vi "RT main.vi"() -> ()   [LabVIEW 2017]
doc: "This example demonstrates how to acquire a continuous amount of data (Waveform) using the DAQ device's internal clock. It also shows how to synchronize two devices for different device families (E Series, S Series, M Series, X Series, DSA, and SC Express), to simultaneously acquire the data.\n\nFor instructions on how to connect your signals to the DAQ device, refer to your device documentation."
uses:
  <vilib>/addons/_NISVFA/_Shared subVIs/Controls/svc_Engineering Units Text Ring.ctl
  <vilib>/addons/_NISVFA/_Shared subVIs/Controls/svc_Weighting Filter Text Ring.ctl
  typedefs/Data.ctl
  <vilib>/Utility/error.llb/DialogType.ctl
  <vilib>/DAQmx/read.llb/DAQmx Read (Analog 1D Wfm NChan NSamp).vi
  <vilib>/Analysis/baseanly.llb/Mean (DBL).vi
  <vilib>/DAQmx/read.llb/DAQmx Read (Analog Wfm 1Chan NSamp).vi
  <vilib>/addons/Sound and Vibration/svt_Calibration/SVL Scale Voltage to EU (1 Ch).vi
  <vilib>/DAQmx/read.llb/DAQmx Read (Analog DBL 1Chan 1Samp).vi
  <extravilib>/ChannelInstances/Stream-a[.](bool)/Read With Abort.vi
  <extravilib>/ChannelInstances/Stream-t'Data.ctl'/Read With Abort.vi
  <extravilib>/ChannelInstances/Stream-a[.](bool)/Write With Abort.vi
  <vilib>/addons/_NISVFA/_Shared subVIs/Common/svc_Set SV Channel Info.vi
  <extravilib>/ChannelInstances/Stream-t'Data.ctl'/Write With Abort.vi
  <extravilib>/ChannelInstances/Stream-a[.](bool)/EndpointRead.vi
  <extravilib>/ChannelInstances/Stream-t'Data.ctl'/EndpointRead.vi
  <extravilib>/ChannelInstances/Stream-a[.](bool)/Endpoint.vi
  <vilib>/addons/_NISVFA/_Shared subVIs/Common/svc_Set SV Channel Info (variant).vi
  <extravilib>/ChannelInstances/Stream-t'Data.ctl'/Endpoint.vi
  <vilib>/addons/_NISVFA/_Shared subVIs/Common/SVL Set dB Reference (variant).vi
  <vilib>/DAQmx/create/channels.llb/DAQmx Create Channel (AI-Voltage-Basic).vi
  <vilib>/DAQmx/configure/timing.llb/DAQmx Timing (Sample Clock).vi
  <vilib>/DAQmx/create/channels.llb/DAQmx Create Channel (AI-Temperature-Thermocouple).vi
  <vilib>/httpClient/POSTBuffer.vi
  <extravilib>/ChannelInstances/Stream-a[.](bool)/Instantiate.vi
  <extravilib>/ChannelInstances/Stream-a[.](bool)/)Channel.vi
  <resource>/ChannelSupport/_ChannelSupport/WaitIfNeeded.vi
  <extravilib>/ChannelInstances/Stream-t'Data.ctl'/Instantiate.vi
  <extravilib>/ChannelInstances/Stream-t'Data.ctl'/)Channel.vi
  <vilib>/Skyline/File/File/Send File.vi
  <vilib>/DAQmx/miscellaneous.llb/DAQmx Fill In Error Info.vi
  <vilib>/addons/Sound and Vibration/Order Analysis/Tach Process/OAT Analog Tacho Process (1 Tacho).vi
  <vilib>/addons/_NISVFA/_Shared subVIs/Common/svc_Engineering Units to Unit Label.vi
  <vilib>/addons/_NISVFA/_Shared subVIs/Common/svc_Compute Scale Factor to Convert V to EU.vi
  <vilib>/addons/_NISVFA/_Shared subVIs/Common/svc_Compute Scale Factor to Convert C to EU.vi
  <vilib>/addons/_NISVFA/_Shared subVIs/Common/svc_Set dB ref if Pascal.vi
  <vilib>/addons/_NISVFA/_Shared subVIs/Common/svc_Caller VI Returned in Error Source.vi
  <vilib>/addons/Sound and Vibration/svt_Level/SVL Running RMS Level (1 Ch).vi
  <vilib>/addons/Sound and Vibration/svt_Calibration/SoundVib_Calibration.lvlib
  <vilib>/addons/Sound and Vibration/svt_Level/SoundVib_VibrationLevel.lvlib
  <vilib>/addons/Sound and Vibration/Order Analysis/Tach Process/SoundVib_TachProcess.lvlib
  <vilib>/Analysis/NI_AALBase.lvlib
  <vilib>/httpClient/LabVIEWHTTPClient.lvlib
  <vilib>/NI_Real-Time Target Support.lvlib
  <extravilib>/ChannelInstances/Stream-t'Data.ctl'.lvlib
  <extravilib>/ChannelInstances/Stream-a[.](bool).lvlib
  <vilib>/Skyline/File/File/NI Skyline File.lvclass
panel:
  out "running RMS":dbl=nan format="%.6f"
  out "network disconnected":T1[](array[typedef]) {"RMS" format="%0.6f"; "RPM" format="%0.2f"; "Voltage" format="%0.2f"; "Current" format="%0.2f"; "Temperature" format="%0.2f"}
  in  "Write to TDMS?":bool
  out "network connected":T1 {"RMS" format="%0.6f"; "RPM" format="%0.2f"; "Voltage" format="%0.2f"; "Current" format="%0.2f"; "Temperature" format="%0.2f"}
  out "Y":bool
  in  "Buttoon 1":bool
  in  "Button 2":bool
  in  "Button 3":bool
  in  "Ipad 2":bool
  in  "Ipad 3":bool
  in  "Ipad 1":bool
  out "Valve":bool[](array[boolean])
  out "X":bool
  out "JSON":string
  in  "integration time [s]":dbl=1.0
  out "Temp.":dbl format="%0.2f"
  out "Current":dbl format="%0.2f"
  out "Voltage":dbl format="%0.2f"
  out "RPM mean":dbl format="%0.2f"
  out "Motor Voltage & Current":waveform(dbl)[](graph)
  in  "Vibration Channel Info":T4={"sensor sensitivity"=1000.0, "engineering units"=1, "dB reference"=1.0, "custom label"="EU", "weighting filter"=0, "pregain"=0.0} {"pregain" format="%.2f"; "weighting filter" items=["Linear", "A-weighting", "B-weighting", "C-weighting", "ITU-R 468-4", "Dolby", "CCITT", "C-message", "Wb", "Wc", "Wd", "We", "Wf", "Wh", "Wj", "Wk", "Wm", "AES17 20 kHz lowpass", "AES17 40 kHz lowpass", "AES17 20 kHz highpass", "AES17 40 kHz highpass"]; "dB reference" format="%^.1e"; "engineering units" items=["custom..."=0, "V"=1, "A"=21, "C"=30, "pC"=31, "s"=32, "-"=29, "Pa"=2, "N"=20, "g"=3, "m/s^2"=4, "m/s"=5, "m"=6, "mm/s"=12, "mm"=13, "micron/s"=14, "micron"=15, "in/s^2"=7, "in/s"=8, "in"=9, "mil/s"=10, "mil"=11, "rad/s^2"=16, "rad/s"=17, "rad"=18, "deg/s^2"=26, "deg/s"=27, "deg"=28, "RPM"=22, "cycle/s^2"=23, "Hz"=24, "cycle"=25, "strain"=19]; "sensor sensitivity" format="%#_5f"}
  in  "Acquire Stop":bool
  in  "CJC Value":dbl=25.0 format="%0.2f"
  in  "CJC Source":i32(ring)=10116 items=["Built-In"=10200, "Constant Value"=10116, "Channel"=10113]
  in  "Thermocouple Type":i32(ring)=10073 items=["J"=10072, "K"=10073, "N"=10077, "R"=10082, "S"=10085, "T"=10086, "B"=10047, "E"=10055]
  in  "Units":i32(ring)=10143 items=["Deg C"=10143, "Deg F"=10144, "Kelvins"=10325, "Deg R"=10145, "From Custom Scale"=10065]
  out "Thermocouple waveform":dbl(graph)
  in  "Motor Voltage & Current & RPM Sample":i32=5120
  in  "Motor Voltage & Current & RPM Sample Rate":dbl=25600.0
  in  "Thermocouple":tag="Mod3/ai1"
  out "Vibration":waveform(dbl)(graph)
  in  "Vibration Sample":i32=5120
  in  "Vibration Sample Rate":dbl=25600.0
  in  "Motor Voltage &Current& RPM":tag="Mod2/ai0:2"
  in  "Vibration":tag="Mod1/ai0"
  # "Vibration Settings"
  # "Vibration"
  # "Motor Voltage & Current & RPM"
  # "Motor Voltage & current & RPM Settings"
  # "Temperature"
  # "Tempearture"
  # "Thermocouple Settings"
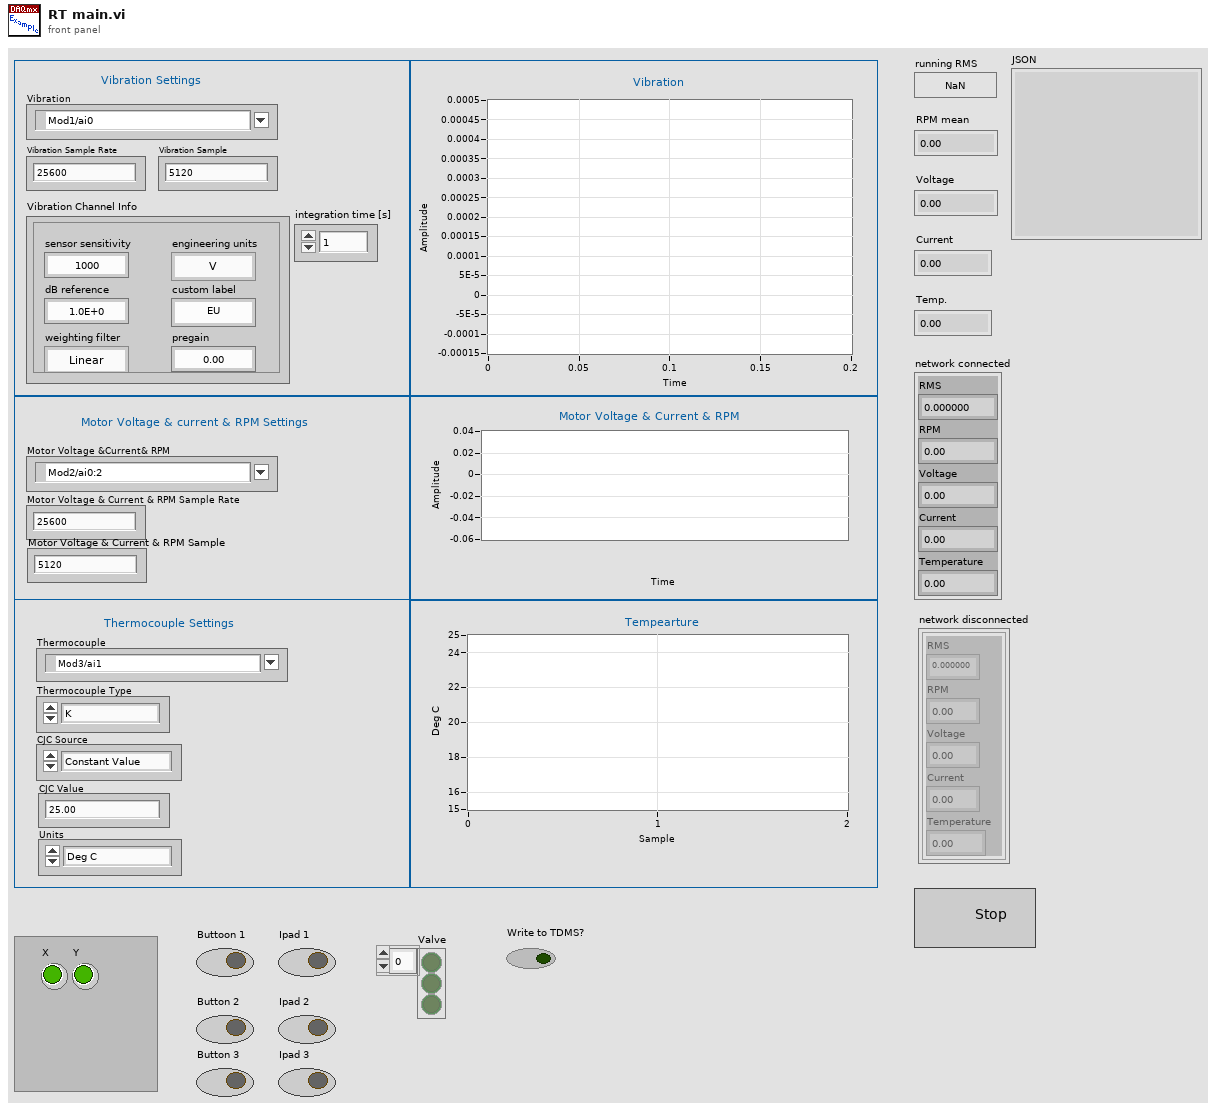
[diagram p1: front panel]
types:
  T1 = typedef "Data.ctl" = cluster{"RMS":dbl, "RPM":dbl, "Voltage":dbl, "Current":dbl, "Temperature":dbl}
  T2 = typedef "svc_Engineering Units Text Ring.ctl" = u16
  T3 = typedef "svc_Weighting Filter Text Ring.ctl" = u16
  T4 = cluster{"sensor sensitivity":dbl, "engineering units":T2, "dB reference":dbl, "custom label":string, "weighting filter":T3, "pregain":dbl}
  T5 = enum16{"open", "open or create", "create or replace", "create", "open (read-only)"}
  T6 = typedef "DialogType.ctl" = u16
  T7 = typedef "SoundVib_TachProcess.lvlib/speed profile.ctl" = cluster{"time [s]":dbl[], "speed [RPM]":dbl[]}
  T8 = typedef "Stream-t'Data.ctl'.lvlib/)Channel.ctl" = refnum<queue>
  T9 = typedef "Stream-a[.](bool).lvlib/)Channel.ctl" = refnum<queue>
  T10 = typedef "LabVIEWHTTPClient.lvlib/ClientHandle.ctl" = refnum<k1>
  T11 = cluster{"RMS":string, "RPM":string, "Voltage":string, "Current":string, "Temperature":string}
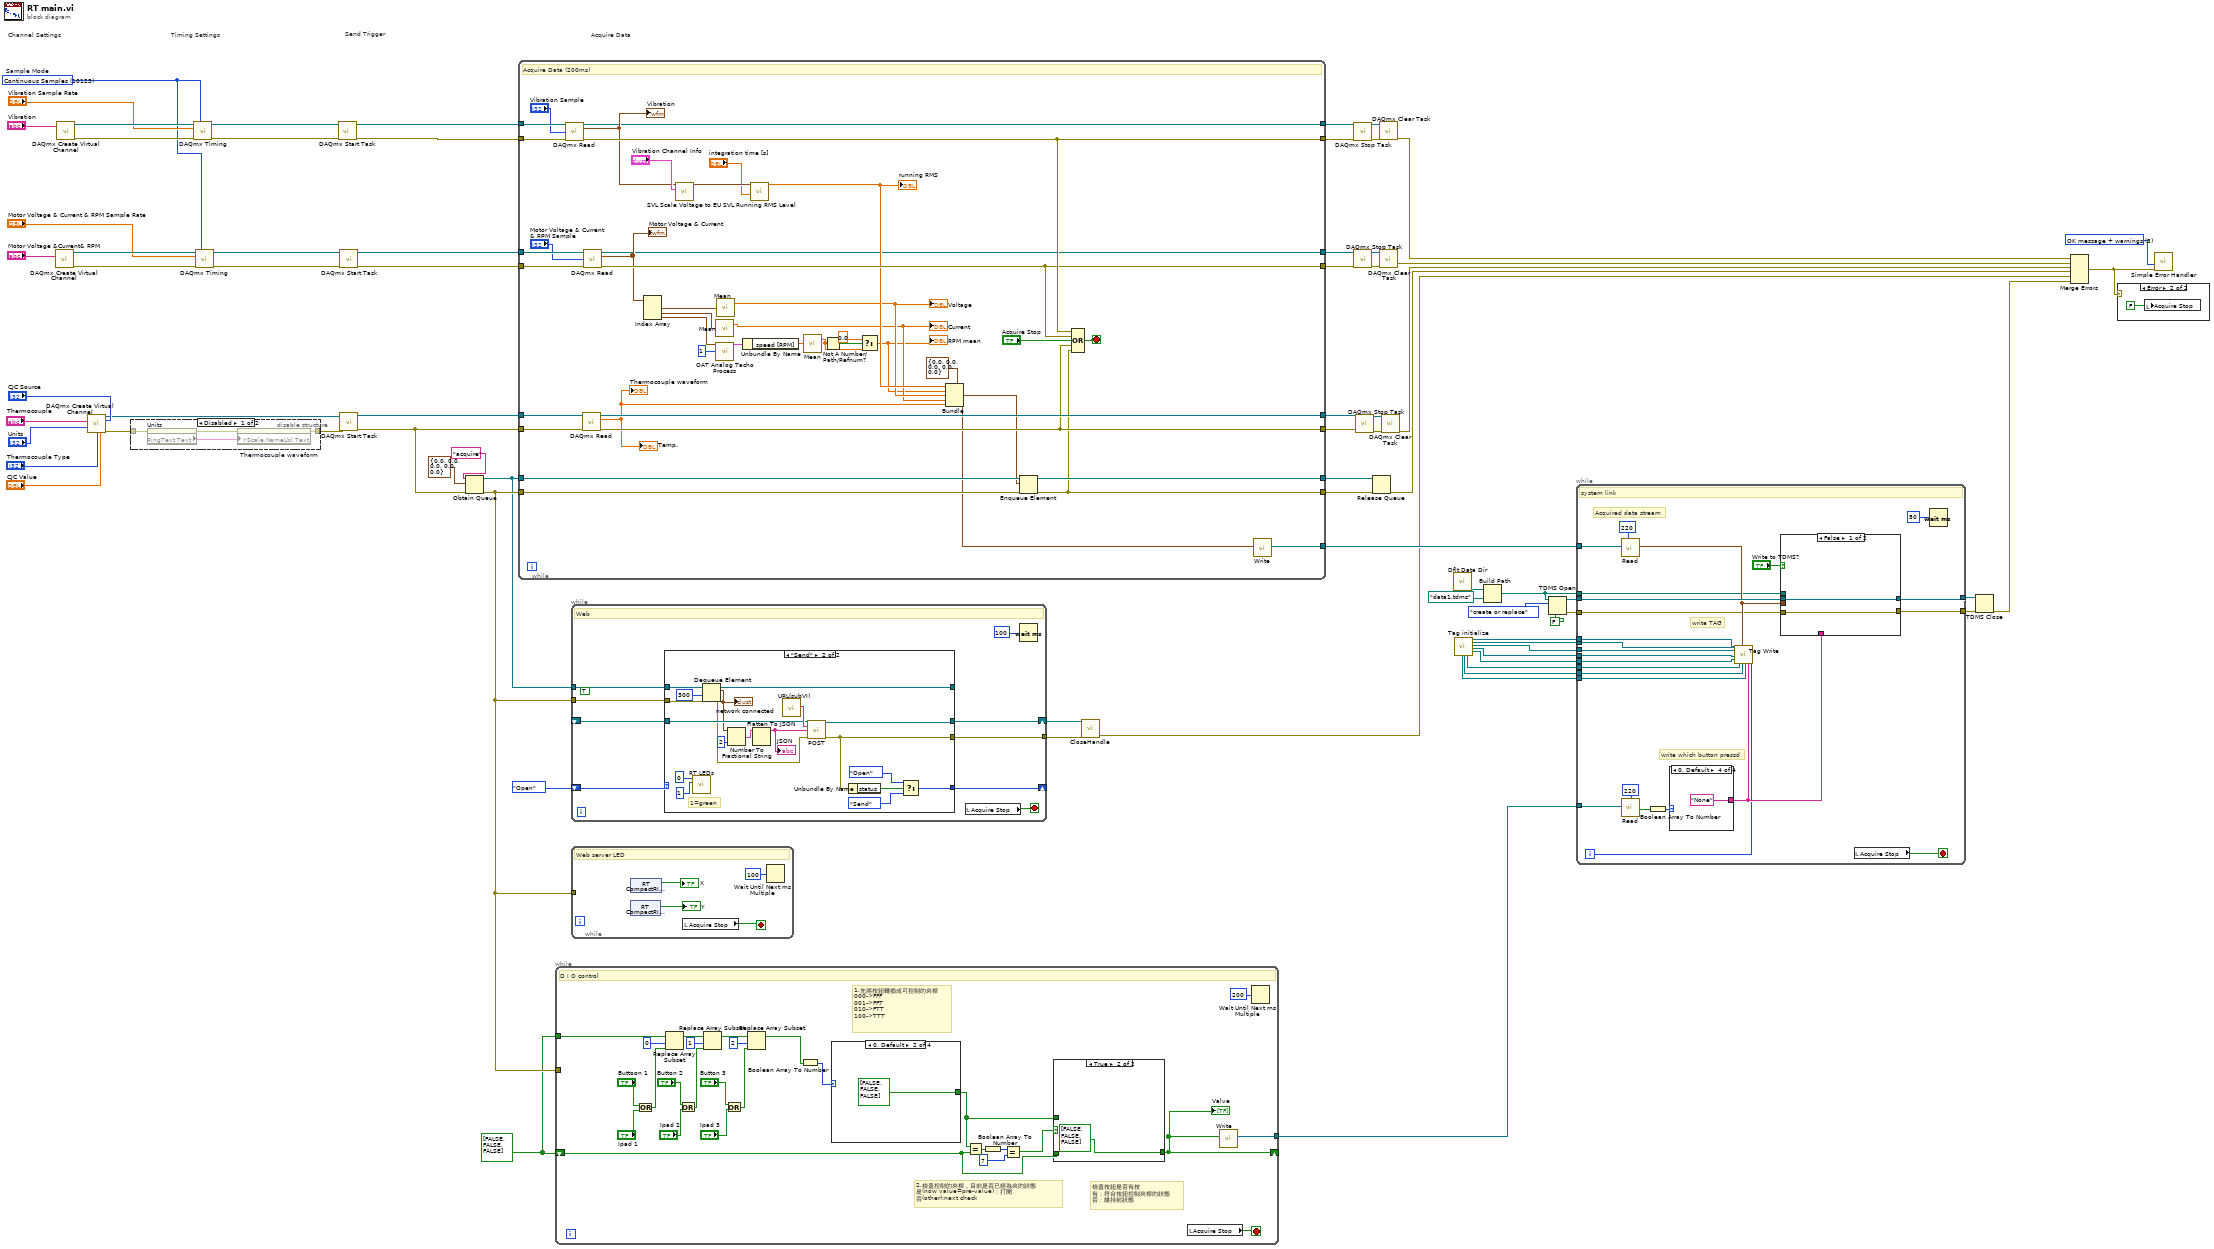
[diagram p0: block diagram]
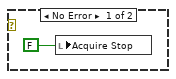
[diagram p2: hidden frame]
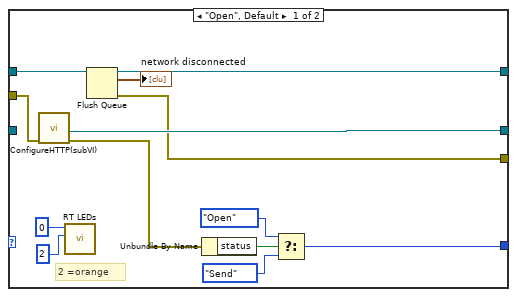
[diagram p3: hidden frame]
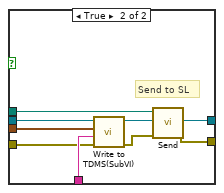
[diagram p4: hidden frame]
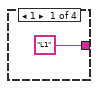
[diagram p5: hidden frame]
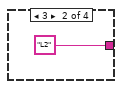
[diagram p6: hidden frame]
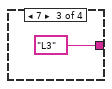
[diagram p7: hidden frame]
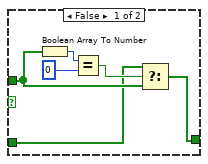
[diagram p8: hidden frame]
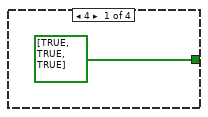
[diagram p9: hidden frame]
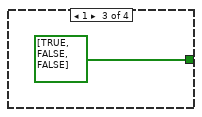
[diagram p10: hidden frame]
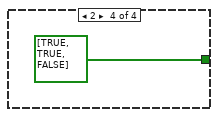
[diagram p11: hidden frame]
diagram:
  w25 = bool[] [FALSE, FALSE, FALSE]
  w54 = T6 3 items=["no dialog", "OK message", "continue or stop message", "OK message + warnings", "continue/stop + warnings"] ("type of dialog (OK msg:1)")
  w53 = 10123 items=["Finite Samples"=10178, "Continuous Samples"=10123, "Hardware Timed Single Point"=12522]  # Sample Mode
  # "Send Trigger"
  # "Acquire Data"
  # "Timing Settings"
  # "Channel Settings"
  n1 = call-poly <vilib>:"DAQmx Create Virtual Channel.vi"("physical channels"="Motor Voltage &Current& RPM") -> ("task out"=w57:refnum<k21>, "error out"=w59:errorcluster)  [unwired: 13 in]
  n2 = call-poly <vilib>:"DAQmx Create Virtual Channel.vi"("physical channels"="Vibration") -> ("task out"=w61:refnum<k21>, "error out"=w60:errorcluster)  [unwired: 13 in]
  n3 = call-poly <vilib>:"DAQmx Create Virtual Channel.vi"("physical channels"="Thermocouple", "cjc source"="CJC Source", "units"="Units", "thermocouple type"="Thermocouple Type", "cjc value"="CJC Value") -> ("task out"=w38:refnum<k21>, "error out"=w40:errorcluster)  [unwired: 9 in]
  n4 = disable-structure shown="Disabled" {
    disable-tunnel: w40 -> [w80 w81]
    disable-tunnel: [w77 w81] -> w37
    frame Disabled {
      n5 = property on="Units" class="Ring (strict)"(error in=w80) -> (error out=w78:errorcluster, "RingText.Text"=w79:string)  [unwired: 1 in, 1 out]
      n6 = property on="Thermocouple waveform" class="WFChart (strict)"(error in=w78, "YScale.NameLbl.Text"=w79) -> (error out=w77:errorcluster)  [unwired: 1 in, 1 out]
    }
    frame Enabled {
    }
  }
  n7 = call-poly <vilib>:"DAQmx Timing.vi"("task/channels in"=w61, "sample mode"=w53, "rate"="Vibration Sample Rate", "error in"=w60) -> ("task out"=w33:refnum<k21>, "error out"=w51:errorcluster)  [unwired: 10 in]
  n8 = call-poly <vilib>:"DAQmx Timing.vi"("task/channels in"=w57, "sample mode"=w53, "rate"="Motor Voltage & Current & RPM Sample Rate", "error in"=w59) -> ("task out"=w58:refnum<k21>, "error out"=w56:errorcluster)  [unwired: 10 in]
  n9 = call <vilib>:"DAQmx Start Task.vi"("task/channels in"=w33, "error in"=w51) -> ("task out"=w76:refnum<k21>, "error out"=w75:errorcluster)  [unwired: 12 in]
  n10 = call <vilib>:"DAQmx Start Task.vi"("task/channels in"=w58, "error in"=w56) -> ("task out"=w74:refnum<k21>, "error out"=w73:errorcluster)  [unwired: 12 in]
  n11 = call <vilib>:"DAQmx Start Task.vi"("task/channels in"=w38, "error in"=w37) -> ("task out"=w50:refnum<k21>, "error out"=w32:errorcluster)  [unwired: 12 in]
  n12 = Obtain Queue(name (unnamed)="acquire", element data type=T1 {"RMS"=0.0, "RPM"=0.0, "Voltage"=0.0, "Current"=0.0, "Temperature"=0.0} ("Data"), error in (no error)=w32) -> (queue out=w1:refnum<queue>, error out=w31:errorcluster)  [unwired: 2 in, 1 out]
  n13 = while {
    tunnel: w50 -> [w115]
    tunnel: w32 -> [w114]
    tunnel: [w113] -> w47
    tunnel: [w112] -> w46
    tunnel: w1 -> [w84]
    tunnel: [w101] -> w36
    tunnel: [w100] -> w35
    tunnel: w31 -> [w99]
    tunnel: w76 -> [w122]
    tunnel: [w92] -> w72
    tunnel: w74 -> [w119]
    tunnel: [w93] -> w68
    tunnel: w73 -> [w118]
    tunnel: [w117] -> w67
    tunnel: w75 -> [w121]
    tunnel: [w120] -> w71
    tunnel: [w82] -> w29
    stop <- w123 stop-if-true
    # "Acquire Data (200ms)"
    n14 = call-poly <vilib>:"DAQmx Read.vi"("task/channels in"=w122, "number of samples per channel"="Vibration Sample", "error in"=w121) -> ("task out"=w92:refnum<k21>, "data"=w95:waveform(dbl), "error out"=w120:errorcluster)  [unwired: 10 in]
    "Vibration" <- w95
    n15 = call-poly <vilib>:"DAQmx Read.vi"("task/channels in"=w115, "error in"=w114) -> ("task out"=w113:refnum<k21>, "data"=w98:dbl, "error out"=w112:errorcluster)  [unwired: 11 in]
    "Thermocouple waveform" <- w98
    "Temp." <- w98
    n16 = call-poly <vilib>:"DAQmx Read.vi"("task/channels in"=w119, "number of samples per channel"="Motor Voltage & Current & RPM Sample", "error in"=w118) -> ("task out"=w93:refnum<k21>, "data"=w105:waveform(dbl)[], "error out"=w117:errorcluster)  [unwired: 10 in]
    "Motor Voltage & Current" <- w105
    n17 = Index Array(array=w105) -> (element #1=w104:waveform(dbl), element #2=w97:waveform(dbl), element #3=w96:waveform(dbl))  [unwired: 3 in]
    n18 = call-poly <vilib>:"SVL Scale Voltage to EU.vi"("channel info"="Vibration Channel Info", "signal [V]"=w95) -> ("scaled signal [EU]"=w109:waveform(dbl))  [unwired: 7 in, 2 out]
    n19 = call-poly <vilib>:"Mean.vi"("X"=w97) -> ("mean"=w89:dbl)  [unwired: 1 out]
    "Current" <- w89
    n20 = call-poly <vilib>:"OAT Analog Tacho Process.vi"("analog tacho signal"=w96, "pulse/revolution (1)"=1) -> ("speed profile"=w107:T7)  [unwired: 9 in, 4 out]
    n21 = call-poly <vilib>:"Mean.vi"("X"=w104) -> ("mean"=w102:dbl)  [unwired: 1 out]
    "Voltage" <- w102
    n22 = Unbundle By Name(w107) -> ("speed [RPM]"=w106:dbl[])
    n23 = call-poly <vilib>:"SVL Running RMS Level.vi"("integration time [s]"="integration time [s]", "scaled signal [EU]"=w109) -> ("running RMS level [EU rms]"=w103:dbl)  [unwired: 6 in, 3 out]
    "running RMS" <- w103
    n24 = call-poly <vilib>:"Mean.vi"("X"=w106) -> ("mean"=w85:dbl)  [unwired: 1 out]
    n25 = Not A Number/Path/Refnum?(number/path/refnum=w85) -> (NaN/Path/Refnum?=w88:bool)
    n26 = Select(t=0.0, s=w88, f=w85) -> (s? t:f=w86:dbl)
    "RPM mean" <- w86
    n27 = Bundle(cluster=T1 {"RMS"=0.0, "RPM"=0.0, "Voltage"=0.0, "Current"=0.0, "Temperature"=0.0} ("Data"), "RMS"=w103, "RPM"=w86, "Voltage"=w102, "Current"=w89, "Temperature"=w98) -> (w83:T1)
    n28 = Enqueue Element(queue=w84, element=w83, error in (no error)=w99) -> (queue out=w101:refnum<queue>, error out=w100:errorcluster)  [unwired: 1 in, 1 out]
    n29 = Compound Arithmetic op=OR(w120, w117, "Acquire Stop", w112, w100) -> (w123:bool)
    n30 = call <extravilib>:"Write.vi"("element"=w83) -> ("channel"=w82:T8)  [unwired: 8 in, 2 out]
  }
  n31 = while {
    shift-right: [w126] -> _
    shift-left: w25 -> [w128]
    tunnel: w31 -> [_]
    tunnel: w25 -> [w127]
    tunnel: [w125] -> w28
    stop <- w124 stop-if-true
    # "1.先將按鈕轉換成可控制的夾桿\n000->FFF\n001->FFT\n010->FTT\n100->TTT"
    # "檢查按鈕是否有按\n有：符合按鈕控制夾桿的狀態\n否：維持前狀態"
    # "2.檢查控制的夾桿，目前是否已經為夾的狀態\n是(now value=pre-value)：打開\n否(other):next check"
    # "D I O control"
    n32 = Or(x="Buttoon 1", y="Ipad 1") -> (x .or. y?=w143:bool)
    n33 = Replace Array Subset(array=w127, new element=w143, index=0) -> (w149:bool[])
    n34 = Or(x="Button 2", y="Ipad 2") -> (x .or. y?=w137:bool)
    n35 = Replace Array Subset(array=w149, new element=w137, index=1) -> (w148:bool[])
    n36 = Or(x="Button 3", y="Ipad 3") -> (x .or. y?=w136:bool)
    n37 = Replace Array Subset(array=w148, new element=w136, index=2) -> (w129:bool[])
    n38 = Boolean Array To Number(Boolean array=w129) -> (number=w131:u32)
    n39 = case shown="0, Default" w131 {
      tunnel: [bool[] [TRUE, TRUE, TRUE] ("Button") bool[] [FALSE, FALSE, FALSE] ("Button") bool[] [TRUE, FALSE, FALSE] ("Button") bool[] [TRUE, TRUE, FALSE] ("Button")] -> w135
      frame 4 {
      }
      frame 0, Default {
      }
      frame 1 {
      }
      frame 2 {
      }
    }
    n40 = Equal?(x=w135, y=w128) -> (x = y?=w132:bool[])
    n41 = Boolean Array To Number(Boolean array=w132) -> (number=w133:u32)
    n42 = Equal?(x=w133, y=u32 7) -> (x = y?=w134:bool)
    n43 = case shown="True" w134 {
      tunnel: [w151 bool[] [FALSE, FALSE, FALSE] ("Button")] -> w126
      tunnel: w135 -> [w153 _]
      tunnel: w128 -> [w152 _]
      frame False {
        n44 = Boolean Array To Number(Boolean array=w153) -> (number=w155:u32)
        n45 = Equal?(x=w155, y=u32 0) -> (x = y?=w154:bool)
        n46 = Select(t=w152, s=w154, f=w153) -> (s? t:f=w151:bool[])
      }
      frame True {
      }
    }
    "Valve" <- w126
    n47 = local read "Acquire Stop"() -> (w124:bool)
    n48 = call <extravilib>:"Write.vi"("element"=w126) -> ("channel"=w125:T9)  [unwired: 8 in, 2 out]
    n49 = Wait Until Next ms Multiple(millisecond multiple=u32 200) -> ()  [unwired: 1 out]
  }
  n50 = while {
    shift-right: [w169] -> _
    shift-left: enum16{"Open", "Send"}."Open" -> [w170]
    shift-right: [w168] -> w8
    shift-left: _ -> [w167]
    tunnel: [w165] -> w9
    tunnel: w31 -> [w162]
    tunnel: w1 -> [w163]
    stop <- w166 stop-if-true
    (unwired) TRUE ("return elements? (F)")
    # "Web"
    n51 = case shown="\"Send\"" w170 {
      tunnel: [w180 w201] -> w169
      tunnel: w162 -> [w179 w198]
      tunnel: [w178 w194] -> _
      tunnel: [w175 w195] -> w168
      tunnel: w167 -> [_ w196]
      tunnel: [w173 w190] -> w165
      tunnel: w163 -> [w172 w187]
      frame "Open", Default {
        # "2 =orange"
        n52 = call "ConfigureHTTP(subVI).vi"("error in (no error)"=w179) -> ("error out"=w174:errorcluster, "Refnum out"=w175:T10)  [unwired: 9 in]
        n53 = call <vilib>:"RT LEDs.vi"("State"=2, "LED Num"=0) -> ()  [unwired: 4 in, 2 out]
        n54 = Flush Queue(queue=w172) -> (queue out=w178:refnum<queue>, remaining elements=→"network disconnected":T1[], error out=w173:errorcluster)  [unwired: 1 in]
        n55 = Unbundle By Name(w174) -> ("status"=w183:bool)
        n56 = Select(t=enum16{"Open", "Send"}."Open", s=w183, f=enum16{"Open", "Send"}."Send") -> (s? t:f=w180:enum16{"Open", "Send"})
      }
      frame "Send" {
        # "1=green"
        n57 = call <vilib>:"RT LEDs.vi"("State"=1, "LED Num"=0) -> ()  [unwired: 4 in, 2 out]
        n58 = Dequeue Element(queue=w187, timeout in ms (-1)=300, error in (no error)=w198) -> (queue out=w194:refnum<queue>, element=w185:T1, error out=w191:errorcluster)  [unwired: 1 out]
        "network connected" <- w185
        n59 = Number To Fractional String(number=w185, precision (6)=i16 2) -> (F-format string=w184:T11)  [unwired: 2 in]
        n60 = Flatten To JSON(anything=w184) -> (JSON string=w189:string)  [unwired: 2 in, 1 out]
        "JSON" <- w189
        n61 = call "URL(subVI).vi"() -> ("URL"=w197:string)  [unwired: 11 in]
        n62 = call-poly <vilib>:"POST.vi"("client handle"=w196, "url"=w197, "buffer"=w189, "error in (no error)"=w191) -> ("client handle out"=w195:T10, "error out"=w190:errorcluster)  [unwired: 8 in, 2 out]
        n63 = Unbundle By Name(w190) -> ("status"=w202:bool)
        n64 = Select(t=enum16{"Open", "Send"}."Open", s=w202, f=enum16{"Open", "Send"}."Send") -> (s? t:f=w201:enum16{"Open", "Send"})
      }
    }
    n65 = local read "Acquire Stop"() -> (w166:bool)
    n66 = Wait (ms)(milliseconds to wait=u32 100) -> ()  [unwired: 1 out]
  }
  n67 = while {
    tunnel: w31 -> [_]
    stop <- w203 stop-if-true
    # "Web server LED"
    n68 = shared-variable "RT CompactRIO Target \\variable.lvlib\\X"() -> (→"X":bool)  [unwired: 1 in, 1 out]
    n69 = shared-variable "RT CompactRIO Target \\variable.lvlib\\Y"() -> (→"Y":bool)  [unwired: 1 in, 1 out]
    n70 = local read "Acquire Stop"() -> (w203:bool)
    n71 = Wait Until Next ms Multiple(millisecond multiple=u32 100) -> ()  [unwired: 1 out]
  }
  n72 = call <vilib>:"CloseHandle.vi"("client handle"=w8, "error in (no error)"=w9) -> ("error out"=w27:errorcluster)  [unwired: 13 in]
  n73 = call <vilib>:"DAQmx Stop Task.vi"("task/channels in"=w72, "error in"=w71) -> ("task out"=w69:refnum<k21>, "error out"=w70:errorcluster)  [unwired: 12 in]
  n74 = call <vilib>:"DAQmx Stop Task.vi"("task/channels in"=w68, "error in"=w67) -> ("task out"=w65:refnum<k21>, "error out"=w66:errorcluster)  [unwired: 12 in]
  n75 = call <vilib>:"DAQmx Stop Task.vi"("task/channels in"=w47, "error in"=w46) -> ("task out"=w49:refnum<k21>, "error out"=w48:errorcluster)  [unwired: 12 in]
  n76 = Release Queue(queue=w36, error in (no error)=w35) -> (error out=w34:errorcluster)  [unwired: 1 in, 2 out]
  n77 = call <vilib>:"DAQmx Clear Task.vi"("task in"=w69, "error in"=w70) -> ("error out"=w64:errorcluster)  [unwired: 13 in]
  n78 = call <vilib>:"DAQmx Clear Task.vi"("task in"=w65, "error in"=w66) -> ("error out"=w3:errorcluster)  [unwired: 13 in]
  n79 = call <vilib>:"DAQmx Clear Task.vi"("task in"=w49, "error in"=w48) -> ("error out"=w45:errorcluster)  [unwired: 13 in]
  n80 = call <vilib>:"Dflt Data Dir.vi"() -> ("App:Default Data Directory"=w23:path)
  n81 = call "Tag initialize.vi"() -> ("Alarm tag"=w4:refnum<class "NI Skyline Tag.lvclass">, "Table tag"=w6:refnum<class "NI Skyline Tag.lvclass">, "Button tag"=w10:refnum<class "NI Skyline Tag.lvclass">, "RMS tag"=w14:refnum<class "NI Skyline Tag.lvclass">, "RPM tag"=w15:refnum<class "NI Skyline Tag.lvclass">, "Voltage tag"=w18:refnum<class "NI Skyline Tag.lvclass">, "Current Tag"=w17:refnum<class "NI Skyline Tag.lvclass">, "Temper tag"=w16:refnum<class "NI Skyline Tag.lvclass">)  [unwired: 11 in, 1 out]
  n82 = Build Path(base path=w23, name or relative path=path "data1.tdms" ("file path")) -> (appended path=w13:path)
  n83 = TDMS Open(6:FALSE ("disable buffering? (T)"), 10:T5."create or replace" ("operation"), 11:w13) -> (0:w11:errorcluster, 3:w20:refnum<k34>)  [unwired: 4 in]
  n84 = while {
    tunnel: w29 -> [w231]
    tunnel: w20 -> [w230]
    tunnel: w28 -> [w229]
    tunnel: [w228] -> w19
    tunnel: w18 -> [w227]
    tunnel: w17 -> [w226]
    tunnel: w16 -> [w225]
    tunnel: w15 -> [w221]
    tunnel: w14 -> [w220]
    tunnel: w13 -> [w218]
    tunnel: [w217] -> w12
    tunnel: w11 -> [w216]
    tunnel: w10 -> [w212]
    tunnel: w6 -> [w211]
    tunnel: w4 -> [w209]
    i -> [w208]
    stop <- w215 stop-if-true
    # "Acquired data stream"
    # "write TAG"
    # "write which button pressd"
    # "system link"
    n85 = call <extravilib>:"Read.vi"("timeout in ms (-1)"=220, "channel"=w231) -> ("element"=w224:T1)  [unwired: 5 in, 4 out]
    n86 = call <extravilib>:"Read.vi"("timeout in ms (-1)"=220, "channel"=w229) -> ("element"=w223:bool[])  [unwired: 5 in, 4 out]
    n87 = Boolean Array To Number(Boolean array=w223) -> (number=w222:u32)
    n88 = case shown="0, Default" w222 {
      tunnel: ["L1" "L2" "L3" "None"] -> w210
      frame 1 {
      }
      frame 3 {
      }
      frame 7 {
      }
      frame 0, Default {
      }
    }
    n89 = call "Tag Write.vi"("RMS tag"=w220, "RPM tag"=w221, "Voltage tag"=w227, "Current tag"=w226, "Temper tag"=w225, "Button tag"=w212, "Data"=w224, "Table tag"=w211, "Alarm tag"=w209, "Btuuon Value"=w210, "i"=w208) -> ()  [unwired: 8 in, 1 out]
    n90 = case shown="False" "Write to TDMS?" {
      tunnel: w230 -> [w233 w241]
      tunnel: [w233 w240] -> w228
      tunnel: w224 -> [_ w239]
      tunnel: w210 -> [_ w238]
      tunnel: w218 -> [_ w236]
      tunnel: [w232 w235] -> w217
      tunnel: w216 -> [w232 w234]
      frame False {
      }
      frame True {
        # "Send to SL"
        n91 = call "Write to TDMS(SubVI).vi"("error in (no error)"=w234, "LED state"=w238, "element"=w239, "Refnum in"=w241) -> ("error out"=w237:errorcluster, "Refnum out"=w240:refnum<k34>)  [unwired: 6 in]
        n92 = call-poly <vilib>:"Send.vi"("error in (no error)"=w237, "path"=w236) -> ("error out"=w235:errorcluster)  [unwired: 7 in, 1 out]
      }
    }
    n93 = local read "Acquire Stop"() -> (w215:bool)
    n94 = Wait (ms)(milliseconds to wait=u32 50) -> ()  [unwired: 1 out]
  }
  n95 = TDMS Close(8:w12, 11:w19) -> (0:w26:errorcluster)  [unwired: 1 out]
  n96 = Merge Errors(w64, w3, w45, w34, w27, w26) -> (w5:errorcluster)
  n97 = case shown="Error" w5 {
    frame No Error {
      n98 = local write "Acquire Stop"(FALSE ("Acquire Stop")) -> ()
    }
    frame Error {
      n99 = local write "Acquire Stop"(FALSE ("Acquire Stop")) -> ()
    }
  }
  n100 = call <vilib>:"Simple Error Handler.vi"("type of dialog (OK msg:1)"=w54, "error in (no error)"=w5) -> ()  [unwired: 3 in, 5 out]
